vi "Control_ERD_Loop.vi"(0 "ERD Loop":refnum<queue>, 2 "Command (ERD Loop Control)":T1=enum."Shutdown", 11 "Error In":errorcluster) -> (15 "Error Out":errorcluster)   [LabVIEW 2021]
uses:
  type defs/ERD_Loop_Control_Command.ctl
  type defs/ERD_Data_Loop_Control.ctl
  type defs/ERD_Loop_States.ctl
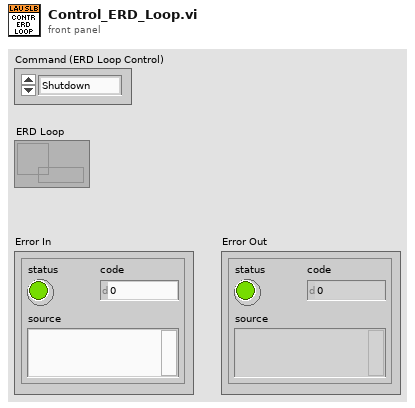
[diagram p1: front panel]
types:
  T1 = typedef "ERD_Loop_Control_Command.ctl" = enum16{"Initialize", "Shutdown"}
  T2 = typedef "ERD_Data_Loop_Control.ctl" = cluster{"Data":variant, "State":T3}
  T3 = typedef "ERD_Loop_States.ctl" = enum16{"Init", "Get Version", "Build ERD Read List", "Read ERDs", "Update UI", "Update Graphs", "Read Faults", "Log Data", "Pause", "Brass Logging", "Shutdown"}
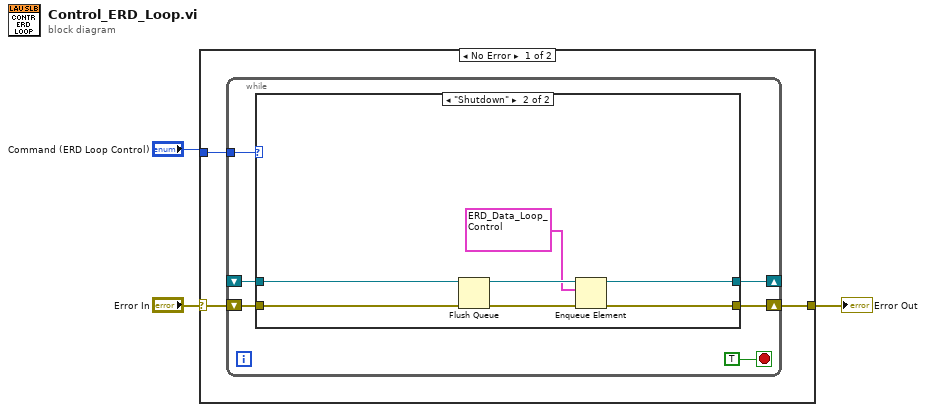
[diagram p0: block diagram]
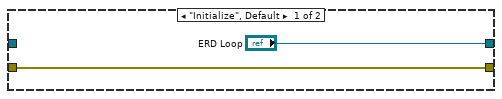
[diagram p2: hidden frame]
diagram:
  n1 = case shown="No Error" "Error In" {
    selector: "Error In" -> [w5 w22]
    tunnel: "Command (ERD Loop Control)" -> [w6 _]
    tunnel: [w4 w22] -> w2
    frame No Error {
      n2 = while {
        tunnel: w6 -> [w12]
        shift-right: [w9] -> w4
        shift-left: w5 -> [w10]
        shift-right: [w8] -> _
        shift-left: _ -> [w7]
        stop <- TRUE stop-if-true
        n3 = case shown="\"Shutdown\"" w12 {
          tunnel: w10 -> [w14 w21]
          tunnel: [w14 w19] -> w9
          tunnel: ["ERD Loop" w18] -> w8
          tunnel: w7 -> [_ w15]
          frame "Initialize", Default {
          }
          frame "Shutdown" {
            n4 = Flush Queue(queue=w15, error in (no error)=w21) -> (queue out=w17:refnum<queue>, error out=w20:errorcluster)  [unwired: 1 out]
            n5 = Enqueue Element(queue=w17, element=T2 {"Data"=variant, "State"=enum."Shutdown"}, error in (no error)=w20) -> (queue out=w18:refnum<queue>, error out=w19:errorcluster)  [unwired: 1 in, 1 out]
          }
        }
      }
    }
    frame Error {
    }
  }
  "Error Out" <- w2
